vi "List Mode - Copy File.vi"(8 "error in (no error)":errorcluster, 9 "Destination File Name":string, 10 "Source File Name":string, 11 "VISA resource name":refnum<visa-resource-name>) -> (0 "error out":errorcluster, 3 "VISA resource name out":refnum<visa-resource-name>)   [LabVIEW 2014, in "Associated Power Technologies 8500 Series.lvlib"]
doc: "Copy file with file name in list mode"
uses:
  <instrlib>/Associated Power Technologies 8500 Series/Associated Power Technologies 8500 Series.lvlib
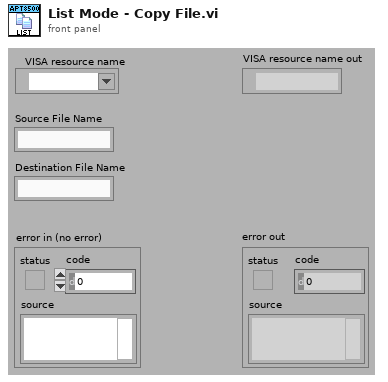
[diagram p1: front panel]
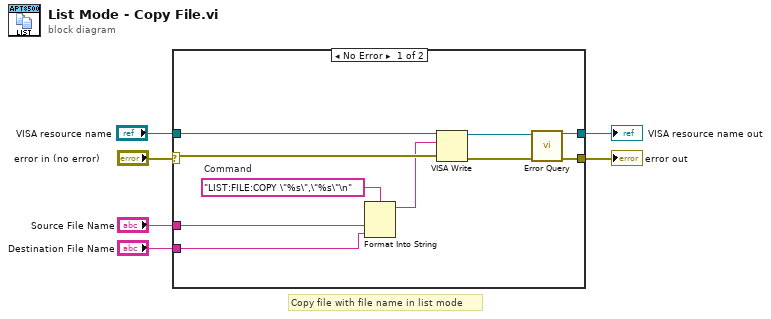
[diagram p0: block diagram]
diagram:
  # "Copy file with file name in list mode"
  n1 = case shown="No Error" "error in (no error)" {
    selector: "error in (no error)" -> [w15 w18]
    tunnel: "VISA resource name" -> [w16 w17]
    tunnel: [w14 w17] -> w6
    tunnel: [w13 w18] -> w5
    tunnel: "Source File Name" -> [w8 _]
    tunnel: "Destination File Name" -> [w7 _]
    frame No Error {
      w9 = "LIST:FILE:COPY \"%s\",\"%s\"\n"  # Command
      n2 = Format Into String(format string=w9, w8, w7) -> (resulting string=w10:string)  [unwired: 2 in, 1 out]
      n3 = VISA Write(VISA resource name=w16, write buffer=w10, error in (no error)=w15) -> (VISA resource name out=w12:refnum<visa-resource-name>, error out=w11:errorcluster)  [unwired: 1 out]
      n4 = call <instrlib>:"Error Query.vi"("VISA resource name"=w12, "error in (no error)"=w11) -> ("VISA resource name out"=w14:refnum<visa-resource-name>, "error out"=w13:errorcluster)  [unwired: 10 in, 2 out]
    }
    frame Error {
    }
  }
  "error out" <- w5
  "VISA resource name out" <- w6
